vi "Selectable bool operation.vi"(2 "Criteria boolean operation":T1, 5 "Criteria x":bool, 9 "Criteria y":bool) -> (8 "x bool operation y.":bool)   [LabVIEW 2011]
uses:
  Boolean operation.ctl
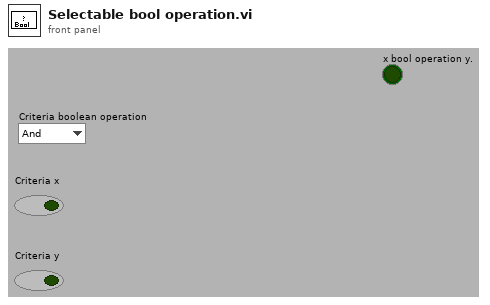
[diagram p1: front panel]
types:
  T1 = typedef "Boolean operation.ctl" = enum16{"And", "Or", "Xor", "Nand", "Nor", "Nxor", "Implies"}
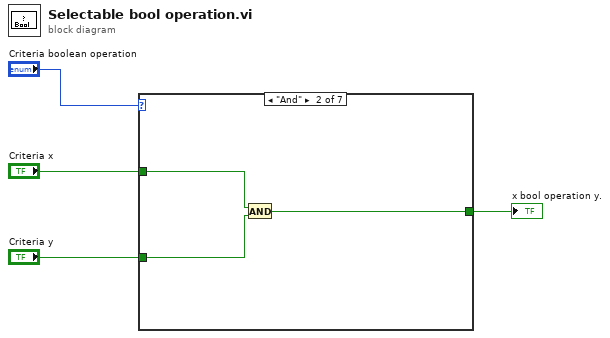
[diagram p0: block diagram]
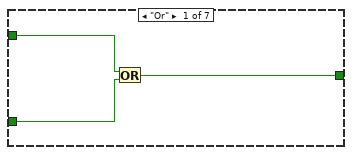
[diagram p2: hidden frame]
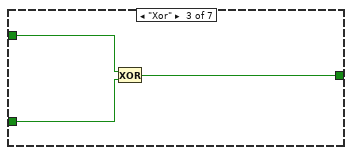
[diagram p3: hidden frame]
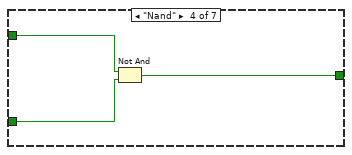
[diagram p4: hidden frame]
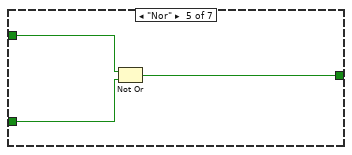
[diagram p5: hidden frame]
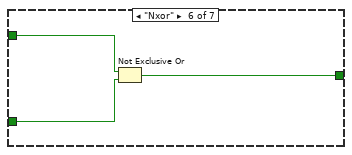
[diagram p6: hidden frame]
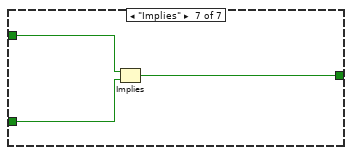
[diagram p7: hidden frame]
diagram:
  n1 = case shown="\"And\"" "Criteria boolean operation" {
    tunnel: "Criteria x" -> [w7 w10 w13 w16 w19 w22 w25]
    tunnel: "Criteria y" -> [w6 w9 w12 w15 w18 w21 w24]
    tunnel: [w5 w8 w11 w14 w17 w20 w23] -> w1
    frame "Or" {
      n2 = Or(x=w7, y=w6) -> (x .or. y?=w5:bool)
    }
    frame "And" {
      n3 = And(x=w10, y=w9) -> (x .and. y?=w8:bool)
    }
    frame "Xor" {
      n4 = Exclusive Or(1:w12, 2:w13) -> (0:w11:bool)
    }
    frame "Nand" {
      n5 = Not And(1:w15, 2:w16) -> (0:w14:bool)
    }
    frame "Nor" {
      n6 = Not Or(1:w18, 2:w19) -> (0:w17:bool)
    }
    frame "Nxor" {
      n7 = Not Exclusive Or(1:w21, 2:w22) -> (0:w20:bool)
    }
    frame "Implies" {
      n8 = Implies(1:w24, 2:w25) -> (0:w23:bool)
    }
  }
  "x bool operation y." <- w1
